vi "Msg.vi"(7 "Actor in":refnum<class "Actor.lvclass">, 11 "Pop Up Msg in":refnum<class "Pop Up Msg.lvclass">) -> (5 "Actor out":refnum<class "Actor.lvclass">)   [LabVIEW 2021, in "Pop Up.lvlib" / "Pop Up Msg.lvclass"]
uses:
  Pop Up Msg.lvclass
  <vilib>/jettl/jettl/Actor/Actor/Actor.lvclass
  Pop Up/Pop Up.lvclass
  c6b198b1-1ebb-4276-964f-c3ad762143cc.vi
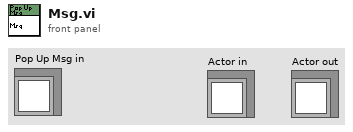
[diagram p1: front panel]
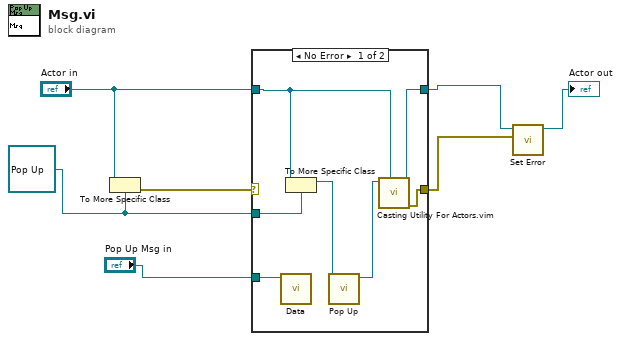
[diagram p0: block diagram]
diagram:
  w3 = refnum<class "Pop Up.lvclass"> refnum ("Pop Up.lvlib:Pop Up.lvclass")
  n1 = To More Specific Class(target class=w3, reference="Actor in") -> (error out=w7:errorcluster)  [unwired: 1 in, 1 out]
  n2 = case shown="No Error" w7 {
    selector: w7 -> [_ w15]
    tunnel: [w13 w16] -> w6
    tunnel: "Actor in" -> [w12 w16]
    tunnel: w3 -> [w14 _]
    tunnel: "Pop Up Msg in" -> [w10 _]
    tunnel: [w11 w15] -> w5
    frame No Error {
      n3 = call "Data.vi"("Pop Up Msg in"=w10) -> ()  [unwired: 11 in]
      n4 = To More Specific Class(target class=w14, reference=w12) -> (specific class reference=w9:refnum<class "Pop Up.lvclass">)  [unwired: 1 in, 1 out]
      n5 = call-dynamic "Pop Up.vi"("Pop Up in"=w9) -> ("Pop Up out"=w8:refnum<class "Pop Up.lvclass">)  [unwired: 10 in]
      n6 = call "Casting Utility For Actors.vim"("type"=w12, "Actor in"=w8) -> ("error out"=w11:errorcluster, "Actor out"=w13:refnum<class "Actor.lvclass">)  [unwired: 8 in]
    }
    frame Error {
    }
  }
  n7 = call-dynamic "Set Error.vi"("Merge"=w5, "Set Error in"=w6) -> ("Set Error out"=→"Actor out":refnum<class "Actor.lvclass">)  [unwired: 9 in]
